vi "Write to File.vi"(8 "error in (no error)":errorcluster, 10 "INI Ref":T1, 11 "Visible Assertion in":refnum<class "Visible Assertion.lvclass">) -> (0 "error out":errorcluster, 2 "INI Ref out":T1, 3 "Visible Assertion out":refnum<class "Visible Assertion.lvclass">)   [LabVIEW 2020, in "MacroAssert.lvlib" / "Visible Assertion.lvclass"]
uses:
  Visible Assertion.lvclass
  Visible Assertion.lvclass/Visible Assertion.ctl
  MacroAssert.lvlib
  <vilib>/Utility/config.llb/NI_LVConfig.lvlib
  <vilib>/Utility/config.llb/Write Key (Boolean).vi
  Control Assertion/Control Assertion.lvclass
  <vilib>/Utility/config.llb/Config Data RefNum.ctl
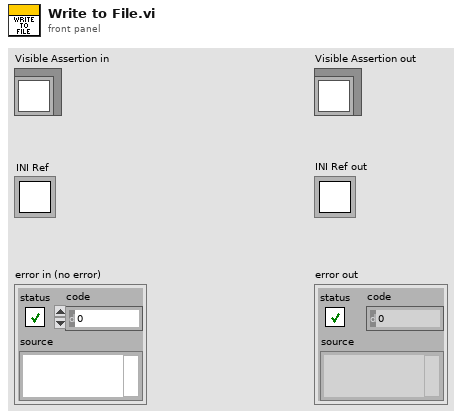
[diagram p1: front panel]
types:
  T1 = typedef "NI_LVConfig.lvlib/Config Data RefNum.ctl" = refnum<k1>
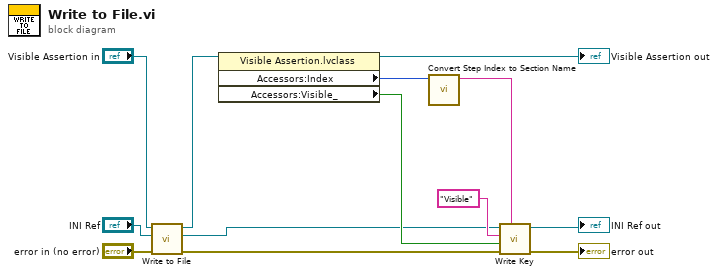
[diagram p0: block diagram]
diagram:
  n1 = call-parent "Write to File.vi"("error in (no error)"="error in (no error)", "INI Ref"="INI Ref", "Control Assertion in"="Visible Assertion in") -> ("error out"=w6:errorcluster, "INI Ref out"=w2:T1, "Control Assertion out"=w5:refnum<class "Visible Assertion.lvclass">)  [unwired: 6 in]
  n2 = property class="Visible Assertion.lvclass"(reference=w5) -> (reference out=→"Visible Assertion out":refnum<class "Visible Assertion.lvclass">, "Accessors:Index"=w9:i32, "Accessors:Visible_"=w7:bool)  [unwired: 1 in, 1 out]
  n3 = call "Convert Step Index to Section Name.vi"("Step Index"=w9) -> ("Section Name"=w8:string)  [unwired: 10 in]
  n4 = call-poly <vilib>:"Write Key.vi"("section"=w8, "error in (no error)"=w6, "value"=w7, "key"="Visible", "refnum"=w2) -> ("error out"=→"error out":errorcluster, "refnum out"=→"INI Ref out":T1)  [unwired: 4 in, 1 out]
